vi "event.vi"() -> ()   [LabVIEW 2013]
panel:
  out "Time":dbl(graph)
  in  "Stop Button":bool
  in  "Mail Button":bool
  out "error out":errorcluster
  out "Boolean":bool
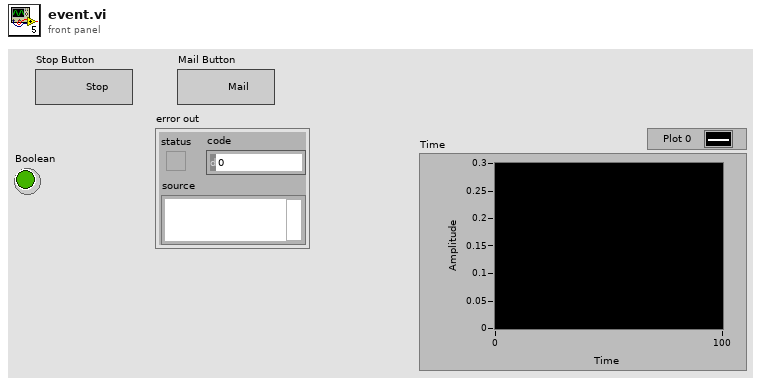
[diagram p1: front panel]
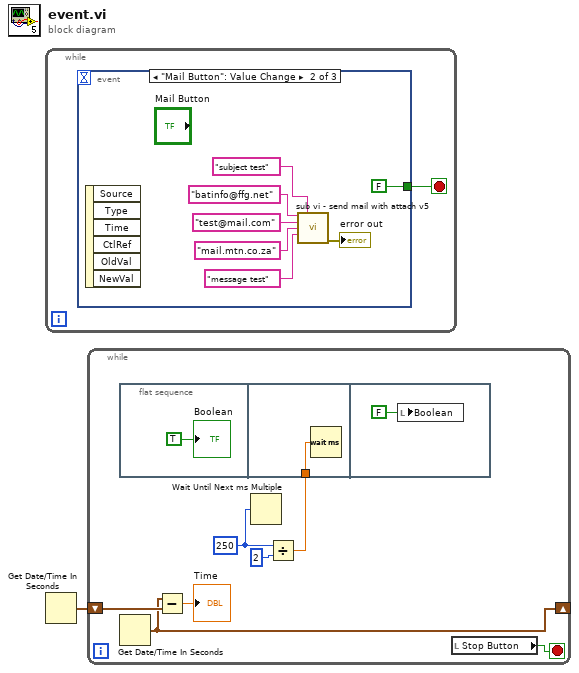
[diagram p0: block diagram]
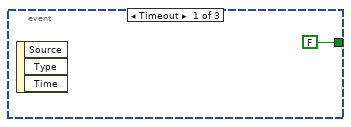
[diagram p2: hidden frame]
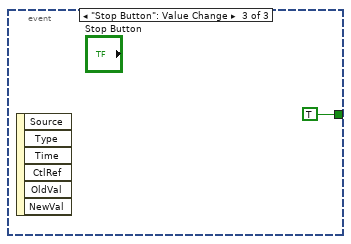
[diagram p3: hidden frame]
diagram:
  n1 = while {
    stop <- w2 stop-if-true
    n2 = event shown="[1] \"Mail Button\": Value Change" {
      selector: _ -> [_ _ _]
      dyn-events: _ -> [_ _ _]
      timeout: _ -> [_ _ _]
      tunnel: [FALSE FALSE TRUE] -> w2
      event Timeout {
        n3 = event-data() -> ()  [unwired: 1 in, 3 out]
      }
      event "Mail Button": Value Change {
        n4 = event-data() -> ()  [unwired: 1 in, 6 out]
        n5 = call "sub vi - send mail with attach v5.vi"("TO:"="batinfo@ffg.net", "subject"="subject test", "from"="test@mail.com", "out going server"="mail.mtn.co.za", "message"="message test") -> ("error out"=→"error out":errorcluster)  [unwired: 10 in]
      }
      event "Stop Button": Value Change {
        n6 = event-data() -> ()  [unwired: 1 in, 6 out]
      }
    }
  }
  n7 = Get Date/Time In Seconds() -> (seconds since 1Jan1904=w1:timestamp)
  n8 = while {
    shift-right: [w16] -> _
    shift-left: w1 -> [w17]
    stop <- w18 stop-if-true
    w14 = u32 250 ("millisecond multiple")
    n9 = flat-sequence {
      tunnel: w12 -> [w20]
      frame #0 {
        "Boolean" <- TRUE ("Boolean")
      }
      frame #1 {
        n10 = Wait (ms)(milliseconds to wait=w20) -> ()  [unwired: 1 out]
      }
      frame #2 {
        n11 = local write "Boolean"(FALSE) -> ()
      }
    }
    n12 = Get Date/Time In Seconds() -> (seconds since 1Jan1904=w16:timestamp)
    n13 = Subtract(x=w16, y=w17) -> (x-y=→"Time":dbl)
    n14 = Wait Until Next ms Multiple(millisecond multiple=w14) -> ()  [unwired: 1 out]
    n15 = Divide(x=w14, y=u32 2) -> (x/y=w12:dbl)
    n16 = local read "Stop Button"() -> (w18:bool)
  }
